vi "SwerveModulePosition_Get.vi"(11 "Swerve Module Position":T2={"Distance"=0.0, "Angle"={"VALUE"=0.0, "COS"=1.0, "SIN"=0.0}} {"Angle"."SIN" format="%13.4f"; "Angle"."COS" format="%13.4f"; "Angle"."VALUE" format="%13.4f"}) -> (0 "Angle Rotation2d":T1={"VALUE"=0.0, "COS"=1.0, "SIN"=0.0} {"SIN" format="%13.4f"; "COS" format="%13.4f"; "VALUE" format="%13.4f"}, 1 "Angle RADIANS":dbl, 3 "Distance M":dbl)   [LabVIEW 2019, in "Trajectory_Library.lvlib"]
doc: "Get the individual position (distance) (meters) and angle (radians) components of the Module Position data cluster.\n\nParmeters:\n - Module Position -- data cluster\n\nReturns:\n - Distance -- Module distance (Meters)\n - Angle -- Module angle (Radians)"
uses:
  Trajectory_Library.lvlib
  TypeDef/ROTATION2D.ctl
  TypeDef/SWERVE_DRIVE_MODULE_POSITION.ctl
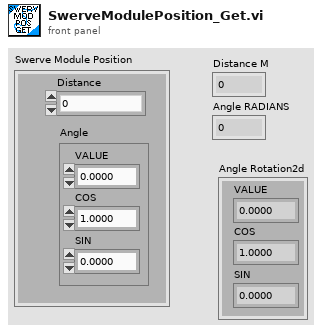
[diagram p1: front panel]
types:
  T1 = typedef "Trajectory_Library.lvlib/ROTATION2D.ctl" = cluster{"VALUE":dbl, "COS":dbl, "SIN":dbl}
  T2 = typedef "Trajectory_Library.lvlib/SWERVE_DRIVE_MODULE_POSITION.ctl" = cluster{"Distance":dbl, "Angle":T1}
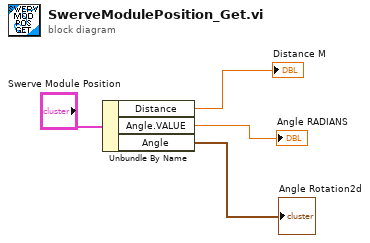
[diagram p0: block diagram]
diagram:
  n1 = Unbundle By Name("Swerve Module Position") -> ("Distance"=→"Distance M":dbl, "Angle.VALUE"=→"Angle RADIANS":dbl, "Angle"=→"Angle Rotation2d":T1)
